vi "GoHome.vi"(8 "error in (no error)":errorcluster, 10 "Axis":enum16{"X", "Y", "Z", "HOM"}(ring), 11 "Arduino_TranslationStage_UI.lvlib:Arduino_Stepper.lvclass":refnum<class "Arduino_Stepper_UI.lvclass">) -> (0 "error out":errorcluster, 3 "Arduino_TranslationStage_UI.lvlib:Arduino_Stepper.lvclass":refnum<class "Arduino_Stepper_UI.lvclass">)   [LabVIEW 2023, in "Arduino_TranslationStage_UI.lvlib" / "Arduino_Stepper_UI.lvclass"]
uses:
  Arduino_Stepper_UI.lvclass
  Arduino_Stepper_UI.lvclass/Arduino_Stepper_UI.ctl
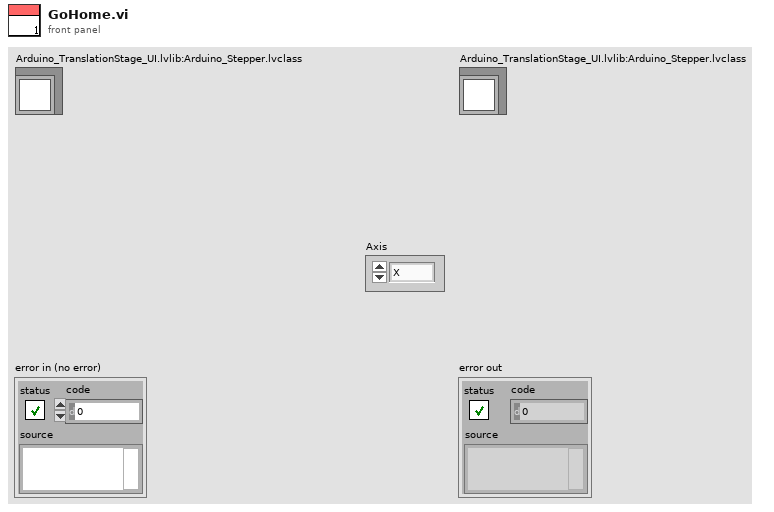
[diagram p1: front panel]
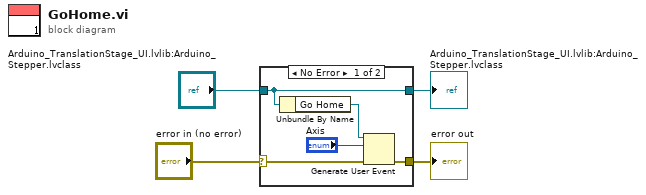
[diagram p0: block diagram]
diagram:
  n1 = case shown="No Error" "error in (no error)" {
    selector: "error in (no error)" -> [w6 w11]
    tunnel: [w5 w11] -> w3
    tunnel: [w9 w10] -> w1
    tunnel: "Arduino_TranslationStage_UI.lvlib:Arduino_Stepper.lvclass" -> [w9 w10]
    frame No Error {
      n2 = Unbundle By Name(w9) -> ("Go Home"=w8:refnum<user-event>)
      n3 = Generate User Event(user event=w8, event data cluster="Axis", error in=w6) -> (error out=w5:errorcluster)  [unwired: 1 in, 1 out]
    }
    frame Error {
    }
  }
  "error out" <- w3
  "Arduino_TranslationStage_UI.lvlib:Arduino_Stepper.lvclass" <- w1
